vi "Update Schedule.vi"(6 "new time":u8, 7 "max geodes in":u8, 8 "max time in":u8, 9 "map in":refnum<data-value>, 10 "stack in":refnum<queue>, 11 "Mine in":refnum<class "Mine.lvclass">) -> (0 "max time out":u8, 1 "map out":refnum<data-value>, 2 "stack out":refnum<queue>, 3 "Mine out":refnum<class "Mine.lvclass">, 5 "max geodes out":u8)   [LabVIEW 2023, in "d19.lvlib" / "Mine.lvclass"]
uses:
  Mine/Mine.lvclass
  <vilib>/Utility/miscctls.llb/LVMapReplaceAction.ctl
  Mine/Mine.lvclass/Mine.ctl
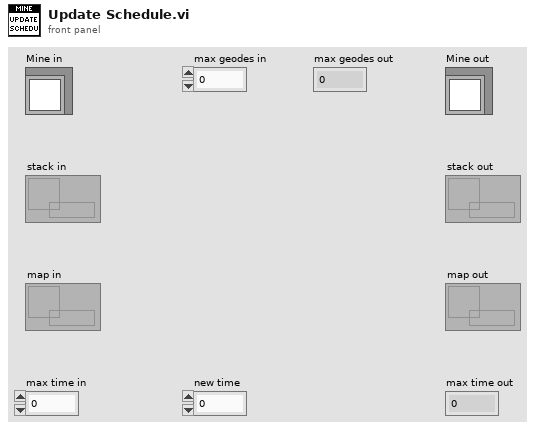
[diagram p1: front panel]
types:
  T1 = typedef "LVMapReplaceAction.ctl" = enum32{"Modify Entry only if found", "Add or Modify Entry", "Delete Entry"}
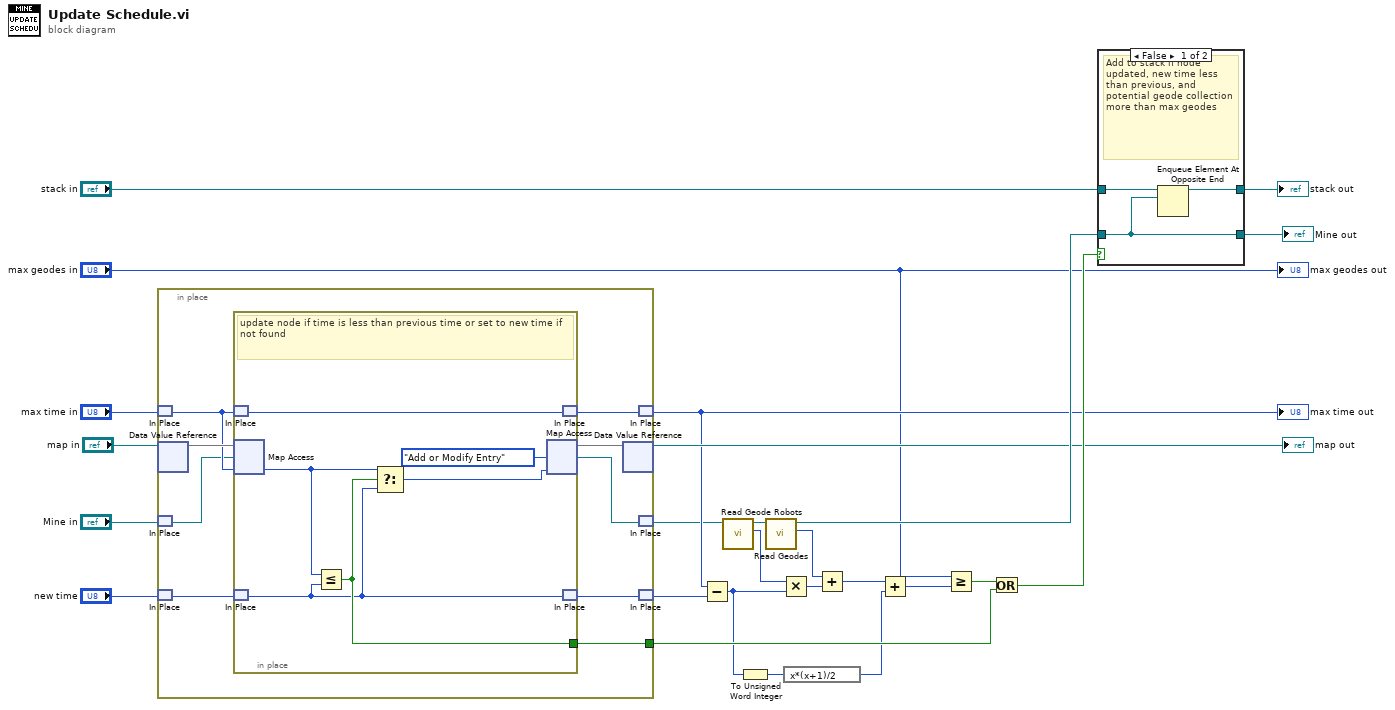
[diagram p0: block diagram]
diagram:
  n1 = in-place {
    in-place-border: [w34] -> w24
    n2 = in-place-match #1("max time in") -> (w31:u8)
    n3 = in-place-dvr #2("map in") -> (w33:map{refnum<class "Mine.lvclass">, u8})  [unwired: 1 out]
    n4 = in-place-match #3("Mine in") -> (w29:refnum<class "Mine.lvclass">)
    n5 = in-place-match #4("new time") -> (w27:u8)
    n6 = in-place {
      in-place-border: [w40] -> w34
      # "update node if time is less than previous time or set to new time if not found"
      n7 = in-place-match #5(w31) -> (w36:u8)
      n8 = in-place-map #6(w33, w29, w31) -> (w38:u8)  [unwired: 1 out]
      n9 = in-place-match #7(w27) -> (w35:u8)
      n10 = Less Or Equal?(x=w38, y=w35) -> (x <= y?=w40:bool)
      n11 = Select(t=w38, s=w40, f=w35) -> (s? t:f=w37:u8)
      n12 = in-place-map #6(w37, LVMapReplaceAction."Add or Modify Entry" ("action")) -> (w32:map{refnum<class "Mine.lvclass">, u8}, w28:refnum<class "Mine.lvclass">)  [unwired: 1 out]
      n13 = in-place-match #5(w36) -> (w30:u8)
      n14 = in-place-match #7(w35) -> (w26:u8)
    }
    n15 = in-place-dvr #2(w32) -> (→"map out":refnum<data-value>)  [unwired: 1 out]
    n16 = in-place-match #1(w30) -> (w11:u8)
    n17 = in-place-match #3(w28) -> (w9:refnum<class "Mine.lvclass">)
    n18 = in-place-match #4(w26) -> (w7:u8)
  }
  "max time out" <- w11
  n19 = Subtract(x=w11, y=w7) -> (x-y=w20:u8)
  n20 = call "Read Geode Robots.vi"("Mine in"=w9) -> ("Geode Robots"=w18:u8, "Mine out"=w19:refnum<class "Mine.lvclass">)  [unwired: 9 in]
  n21 = To Unsigned Word Integer(number=w20) -> (unsigned 16bit integer=w1:u16)
  n22 = call "Read Geodes.vi"("Mine in"=w19) -> ("Geodes"=w5:u8, "Mine out"=w23:refnum<class "Mine.lvclass">)  [unwired: 9 in]
  n23 = Multiply(x=w18, y=w20) -> (x*y=w17:u8)
  n24 = expression code="x*(x+1)/2"(w1) -> (w16:u16)
  n25 = Add(x=w5, y=w17) -> (x+y=w3:u8)
  n26 = Add(x=w3, y=w16) -> (x+y=w15:u16)
  n27 = Greater Or Equal?(x="max geodes in", y=w15) -> (x >= y?=w4:bool)
  n28 = Or(x=w4, y=w24) -> (x .or. y?=w25:bool)
  n29 = case shown="False" w25 {
    tunnel: "stack in" -> [w43 w45]
    tunnel: [w42 w45] -> w22
    tunnel: w23 -> [w41 w44]
    tunnel: [w41 w44] -> w2
    frame False {
      # "Add to stack if node updated, new time less than previous, and potential geode collection more than max geodes"
      n30 = Enqueue Element At Opposite End(queue=w43, element=w41) -> (queue out=w42:refnum<queue>)  [unwired: 2 in, 2 out]
    }
    frame True {
    }
  }
  "stack out" <- w22
  "Mine out" <- w2
  "max geodes out" <- "max geodes in"
